vi "Adjust Cordinates.vi"(8 "error in (no error)":errorcluster, 10 "Coords":T1, 11 "VI in":refnum<vi>) -> (0 "error out":errorcluster, 2 "Coords out":T1)   [LabVIEW 2013, in "Table Manager.lvlib" / "Mapping Column.lvclass"]
uses:
  Mapping Column.lvclass
  <vilib>/Utility/miscctls.llb/LVPoint32TypeDef.ctl
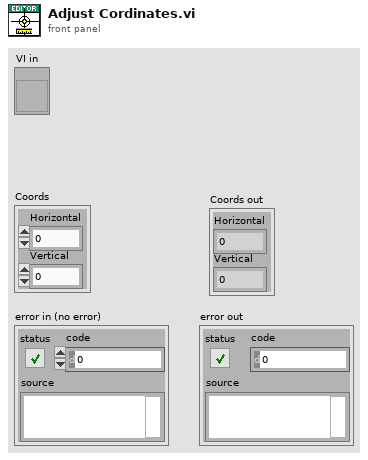
[diagram p1: front panel]
types:
  T1 = typedef "LVPoint32TypeDef.ctl" = cluster{"Horizontal":i32, "Vertical":i32}
  T2 = typedef "LVRectTypeDef.ctl" = cluster{"Left":i16, "Top":i16, "Right":i16, "Bottom":i16}
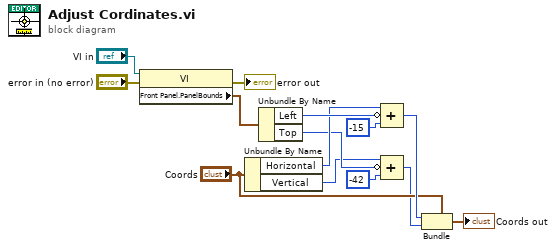
[diagram p0: block diagram]
diagram:
  n1 = property class="VI"(reference="VI in", error in="error in (no error)") -> (error out=→"error out":errorcluster, "Front Panel.PanelBounds"=w10:T2)  [unwired: 1 out]
  n2 = Unbundle By Name("Coords") -> ("Horizontal"=w6:i32, "Vertical"=w4:i32)
  n3 = Unbundle By Name(w10) -> ("Left"=w7:i16, "Top"=w5:i16)
  n4 = Compound Arithmetic op=ADD(w6, invert w7, i16 -15 ("value")) -> (w9:i32)
  n5 = Compound Arithmetic op=ADD(w4, invert w5, i16 -42 ("value 2")) -> (w3:i32)
  n6 = Bundle(cluster="Coords", "Horizontal"=w9, "Vertical"=w3) -> (→"Coords out":T1)
